vi "05.1-4 Read Config File (subVI).vi"(8 "Error In":errorcluster, 11 "Config File In":path) -> (0 "Error Out":errorcluster, 2 "Hardware Settings":T1={"AI Channel"="Multi_I-O/ai0", "Sample Rate"=1000.0, "Samples per Channel"=1000, "AO Channel"="Multi_I-O/ao1"}, 3 "Config File Out":path)   [LabVIEW 2019]
uses:
  05.1 Hardware Settings.ctl
  <vilib>/Utility/config.llb/Read Key (String).vi
  <vilib>/Utility/config.llb/Read Key (Double).vi
  <vilib>/Utility/config.llb/Read Key (I32).vi
  <vilib>/Utility/config.llb/NI_LVConfig.lvlib
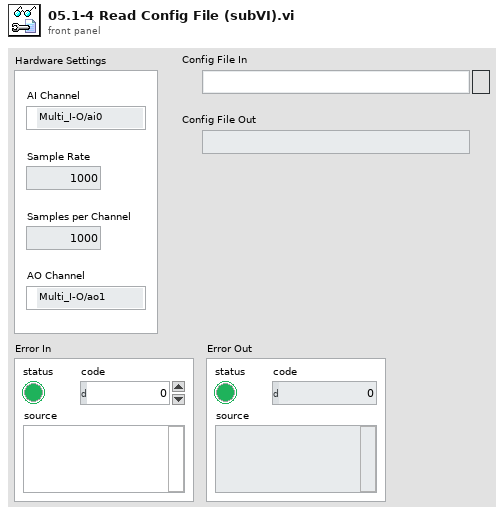
[diagram p1: front panel]
types:
  T1 = typedef "05.1 Hardware Settings.ctl" = cluster{"AI Channel":tag, "Sample Rate":dbl, "Samples per Channel":i32, "AO Channel":tag}
  T2 = typedef "NI_LVConfig.lvlib/Config Data RefNum.ctl" = refnum<k1>
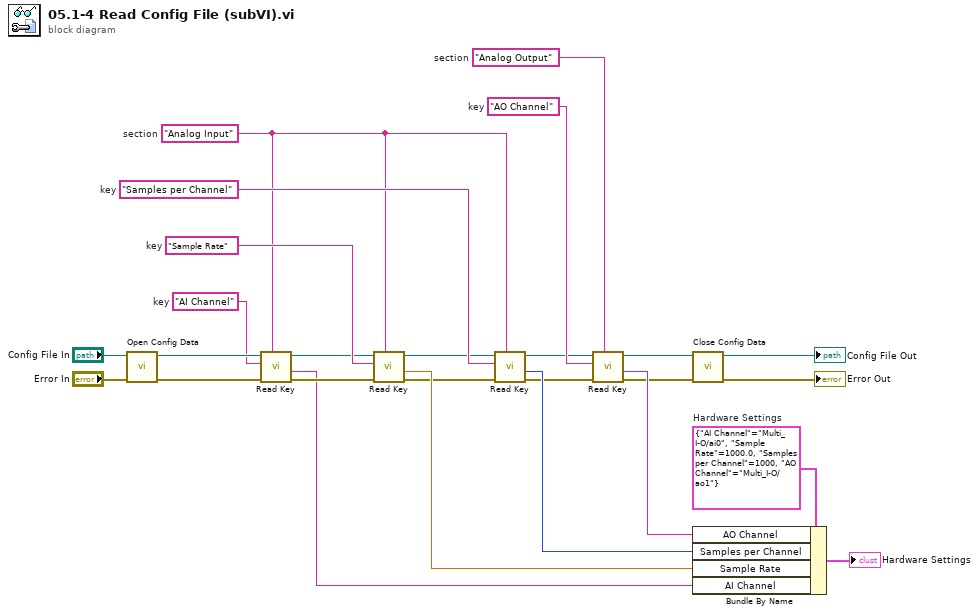
[diagram p0: block diagram]
diagram:
  w14 = "AO Channel"  # key
  w12 = "Analog Output"  # section
  w17 = "Samples per Channel"  # key
  w19 = "Sample Rate"  # key
  w23 = "AI Channel"  # key
  w16 = "Analog Input"  # section
  w26 = T1 {"AI Channel"="Multi_I-O/ai0", "Sample Rate"=1000.0, "Samples per Channel"=1000, "AO Channel"="Multi_I-O/ao1"}  # Hardware Settings
  n1 = call <vilib>:"Open Config Data.vi"("error in (no error)"="Error In", "configuration file path"="Config File In") -> ("error out"=w25:errorcluster, "refnum"=w24:T2)  [unwired: 7 in, 1 out]
  n2 = call-poly <vilib>:"Read Key.vi"("section"=w16, "error in (no error)"=w25, "key"=w23, "refnum"=w24) -> ("error out"=w22:errorcluster, "value"=w21:string, "refnum out"=w8:T2)  [unwired: 4 in, 1 out]
  n3 = call-poly <vilib>:"Read Key.vi"("section"=w16, "error in (no error)"=w22, "key"=w19, "refnum"=w8) -> ("error out"=w18:errorcluster, "value"=w20:dbl, "refnum out"=w7:T2)  [unwired: 4 in, 1 out]
  n4 = call-poly <vilib>:"Read Key.vi"("section"=w16, "error in (no error)"=w18, "key"=w17, "refnum"=w7) -> ("error out"=w13:errorcluster, "value"=w15:i32, "refnum out"=w6:T2)  [unwired: 4 in, 1 out]
  n5 = call-poly <vilib>:"Read Key.vi"("section"=w12, "error in (no error)"=w13, "key"=w14, "refnum"=w6) -> ("error out"=w10:errorcluster, "value"=w11:string, "refnum out"=w9:T2)  [unwired: 4 in, 1 out]
  n6 = call <vilib>:"Close Config Data.vi"("error in (no error)"=w10, "refnum"=w9) -> ("error out"=→"Error Out":errorcluster, "file path"=→"Config File Out":path)  [unwired: 8 in]
  n7 = Bundle By Name(cluster=w26, "AO Channel"=w11, "Samples per Channel"=w15, "Sample Rate"=w20, "AI Channel"=w21) -> (→"Hardware Settings":T1)
